vi "SystemExecOption.vi"() -> ()   [LabVIEW 2023]
panel:
  in  "send":bool
  in  "content":string
  out "spreadsheet string":string
  in  "stop":bool
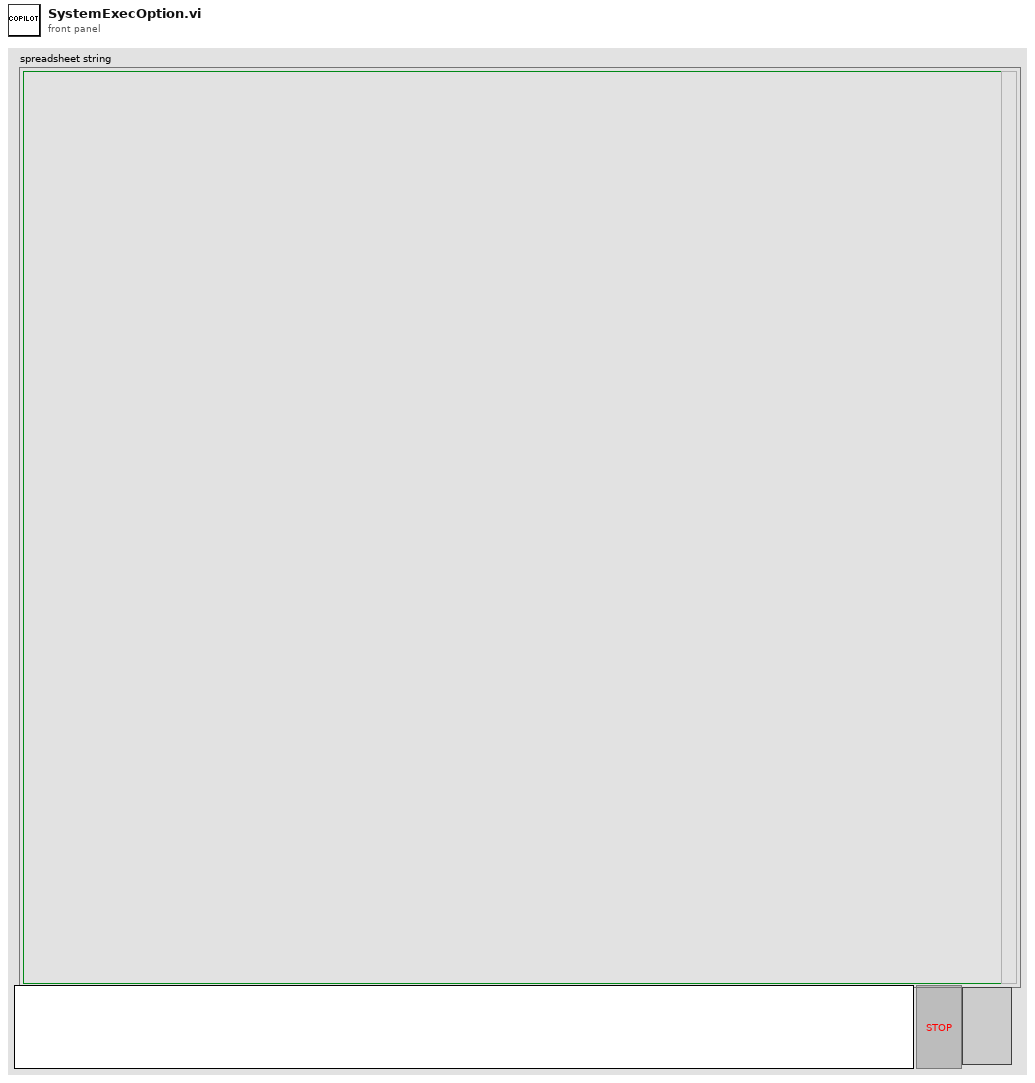
[diagram p1: front panel]
types:
  T1 = cluster{"History":cluster{"role":string, "content":string}[]}
  T2 = cluster{"History":cluster{"role":string, "content":string}[], "content":string}
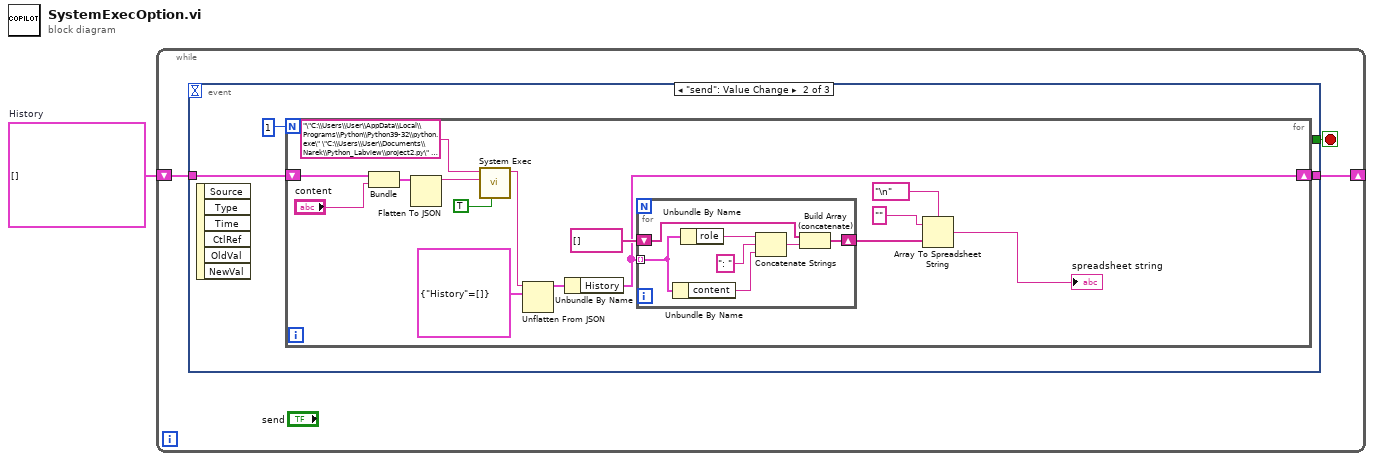
[diagram p0: block diagram]
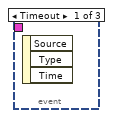
[diagram p2: hidden frame]
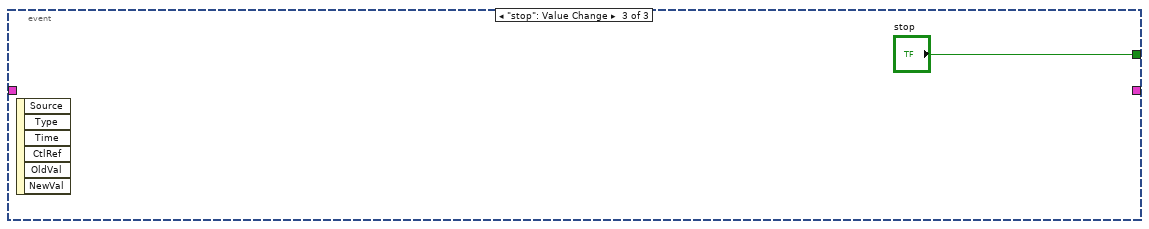
[diagram p3: hidden frame]
diagram:
  w1 = cluster{"role":string, "content":string}[] []  # History
  n1 = while {
    shift-right: [w2] -> _
    shift-left: w1 -> [w3]
    stop <- w4 stop-if-true
    n2 = event shown="[1] \"send\": Value Change" {
      selector: _ -> [_ _ _]
      dyn-events: _ -> [_ _ _]
      timeout: _ -> [_ _ _]
      tunnel: [_ _ "stop"] -> w4
      tunnel: w3 -> [_ w6 _]
      tunnel: [_ w5 _] -> w2
      event Timeout {
        n3 = event-data() -> ()  [unwired: 1 in, 3 out]
      }
      event "send": Value Change {
        n4 = event-data() -> ()  [unwired: 1 in, 6 out]
        n5 = for {
          N: 1 -> [_]
          shift-right: [w13] -> w5
          shift-left: w6 -> [w14]
          n6 = Bundle("History"=w14, "content"="content") -> (w11:T2)  [unwired: 1 in]
          n7 = Flatten To JSON(anything=w11) -> (JSON string=w10:string)  [unwired: 2 in, 1 out]
          n8 = call <vilib>:"System Exec.vi"("run minimized? (F)"=TRUE, "standard input"=w10, "command line"="\"C:\\Users\\User\\AppData\\Local\\Programs\\Python\\Python39-32\\python.exe\" \"C:\\Users\\User\\Documents\\Narek\\Python_Labview\\project2.py\" \"{\\\"History\\\": [], \\\"content\\\": \\\"Hello LabVIEW\\\"}\" ") -> ("standard output"=w8:string)  [unwired: 5 in, 3 out]
          n9 = Unflatten From JSON(JSON string=w8, type and defaults=T1 {"History"=[]} ("output cluster")) -> (value=w12:T1)  [unwired: 5 in, 1 out]
          n10 = Unbundle By Name(w12) -> ("History"=w13:cluster{"role":string, "content":string}[])
          n11 = for {
            tunnel: w13 -> [w24] mode=indexing
            shift-right: [w28] -> w15
            shift-left: string[] [] -> [w29]
            n12 = Unbundle By Name(w24) -> ("content"=w23:string)
            n13 = Unbundle By Name(w24) -> ("role"=w27:string)
            n14 = Concatenate Strings(w27, ": " ("string"), w23) -> (w25:string)
            n15 = Build Array (concatenate)(w29, w25) -> (w28:string[])
          }
          n16 = Array To Spreadsheet String(delimiter (Tab)="\n", array=w15, 3:"" ("format string")) -> (spreadsheet string=→"spreadsheet string":string)
        }
      }
      event "stop": Value Change {
        n17 = event-data() -> ()  [unwired: 1 in, 6 out]
      }
    }
  }
